vi "Center With Gyro Logic.vi"(0 "Angle":dbl, 5 "Face Where?":dbl) -> (4 "Disable Drive":bool, 6 "Too Far to the Right":bool, 10 "Too Far to the Left":bool)   [LabVIEW 2015]
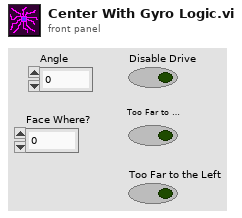
[diagram p1: front panel]
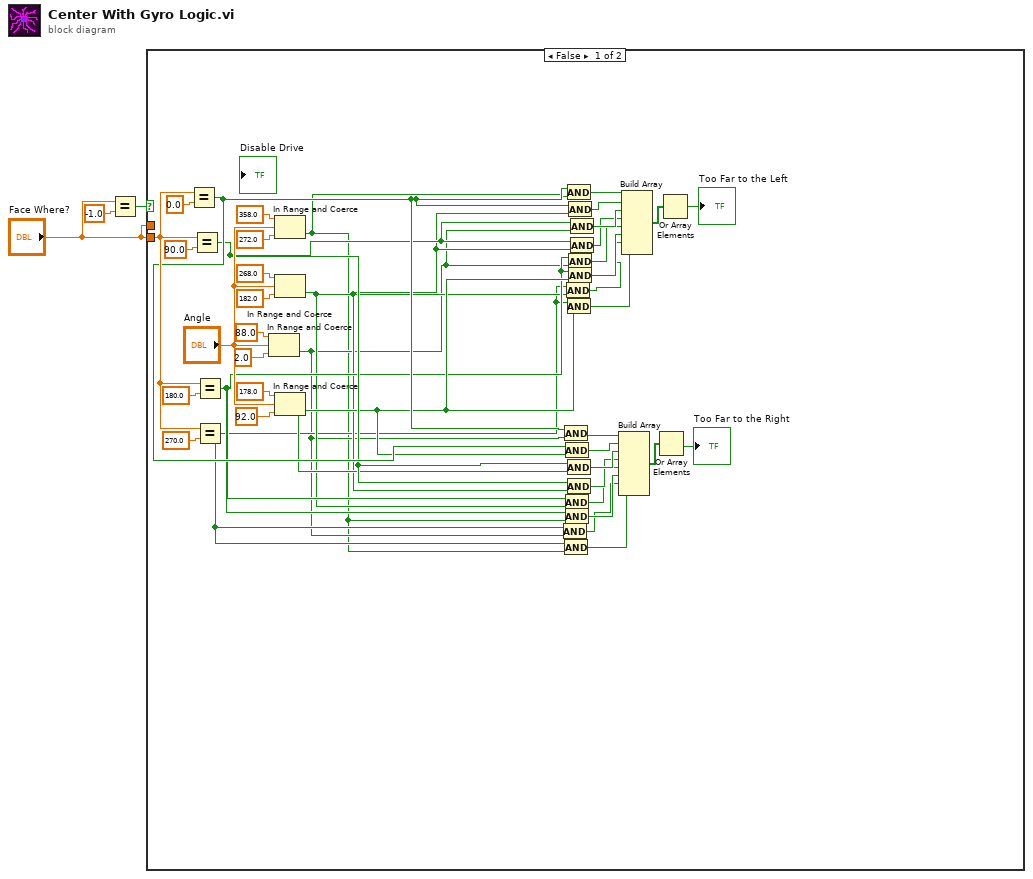
[diagram p0: block diagram]
diagram:
  n1 = Equal?(x="Face Where?", y=-1.0) -> (x = y?=w3:bool)
  n2 = case shown="False" w3 {
    tunnel: "Face Where?" -> [_ _]
    tunnel: "Face Where?" -> [w40 _]
    frame False {
      n3 = Equal?(x=w40, y=0.0) -> (x = y?=w11:bool)
      n4 = Equal?(x=w40, y=90.0) -> (x = y?=w10:bool)
      n5 = Equal?(x=w40, y=180.0) -> (x = y?=w8:bool)
      n6 = Equal?(x=w40, y=270.0) -> (x = y?=w6:bool)
      n7 = In Range and Coerce(upper limit=88.0 ("lower limit"), x="Angle", lower limit=2.0 ("upper limit")) -> (In Range?=w5:bool)  [unwired: 1 out]
      n8 = In Range and Coerce(upper limit=358.0 ("lower limit"), x="Angle", lower limit=272.0 ("upper limit")) -> (In Range?=w4:bool)  [unwired: 1 out]
      n9 = In Range and Coerce(upper limit=268.0 ("lower limit"), x="Angle", lower limit=182.0 ("upper limit")) -> (In Range?=w7:bool)  [unwired: 1 out]
      n10 = In Range and Coerce(upper limit=178.0 ("lower limit"), x="Angle", lower limit=92.0 ("upper limit")) -> (In Range?=w9:bool)  [unwired: 1 out]
      n11 = And(x=w6, y=w5) -> (x .and. y?=w13:bool)
      n12 = And(x=w11, y=w5) -> (x .and. y?=w19:bool)
      n13 = And(x=w6, y=w4) -> (x .and. y?=w12:bool)
      n14 = And(x=w11, y=w9) -> (x .and. y?=w17:bool)
      n15 = And(x=w8, y=w7) -> (x .and. y?=w15:bool)
      n16 = And(x=w8, y=w4) -> (x .and. y?=w14:bool)
      n17 = And(x=w6, y=w7) -> (x .and. y?=w22:bool)
      n18 = And(x=w11, y=w4) -> (x .and. y?=w28:bool)
      n19 = And(x=w6, y=w9) -> (x .and. y?=w21:bool)
      n20 = And(x=w10, y=w9) -> (x .and. y?=w18:bool)
      n21 = And(x=w10, y=w7) -> (x .and. y?=w16:bool)
      n22 = And(x=w11, y=w7) -> (x .and. y?=w27:bool)
      n23 = And(x=w8, y=w5) -> (x .and. y?=w24:bool)
      n24 = And(x=w8, y=w9) -> (x .and. y?=w23:bool)
      n25 = And(x=w10, y=w5) -> (x .and. y?=w26:bool)
      n26 = And(x=w10, y=w7) -> (x .and. y?=w25:bool)
      n27 = Build Array(w19, w17, w18, w16, w15, w14, w13, w12) -> (w20:bool[])
      n28 = Build Array(w28, w27, w26, w25, w24, w23, w22, w21) -> (w29:bool[])
      n29 = Or Array Elements(Boolean array=w20) -> (logical OR=→"Too Far to the Right":bool)
      n30 = Or Array Elements(Boolean array=w29) -> (logical OR=→"Too Far to the Left":bool)
    }
    frame True {
    }
  }
